vi "Fluence in multiple areas.vi"(0 "Analyze Fluence in":refnum<class "Analyze Fluence.lvclass">, 5 "Image in":T2, 7 "Energy":dbl[unit], 11 "error in (no error)":errorcluster) -> (4 "Analyze Fluence out":refnum<class "Analyze Fluence.lvclass">, 6 "Image Dst Out":T2, 8 "Max Fluence J/cm^2":dbl[unit], 10 "fluence infos":T3[](array[typedef]), 15 "error out":errorcluster)   [LabVIEW 2014, in "Analyze.lvlib" / "Analyze Fluence.lvclass"]
uses:
  Analyze Fluence.lvclass
  Fluence Info.ctl
  <vilib>/vision/Image Controls.llb/IMAQ Image.ctl
  Analyze Parameter/Analyze Parameter Fluence/Analyze Parameter Fluence.lvclass
  Analyze Fluence.lvclass/Analyze Fluence.ctl
  <vilib>/vision/NI_Vision_Development_Module.lvlib
  Analyze BaseClass/Analyze BaseClass/Analyze BaseClass.lvclass
panel:
  in  "ROI Descriptor out":T1 {"Contours"."Type" items=["No Selection", "Point", "Line", "Rectangle", "Oval", "Polygon", "Freehand Region", "Annulus", "Unused2", "Unused3", "Broken Line", "Freehand Line", "Rotated Rectangle"]}
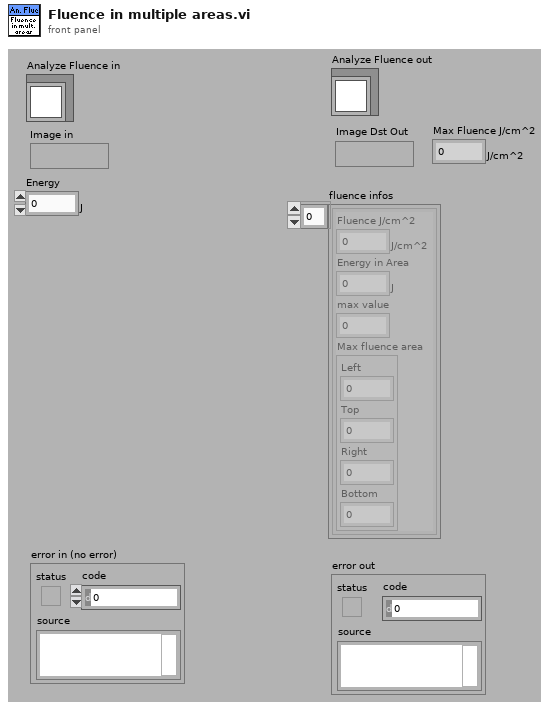
[diagram p1: front panel]
types:
  T1 = typedef "ROI Descriptor" = cluster{"Global Rectangle":i32[], "Contours":cluster{"ID":enum32{"External", "Internal"}, "Type":u32, "Coordinates":i32[]}[]}
  T2 = typedef "IMAQ Image.ctl" = refnum<image>
  T3 = typedef "Analyze.lvlib/Analyze Fluence.lvclass/Fluence Info.ctl" = cluster{"Fluence J/cm^2":dbl[unit], "Energy in Area":dbl[unit], "max value":i64, "Max fluence area":cluster{"Left":i32, "Top":i32, "Right":i32, "Bottom":i32}}
  T4 = typedef "IMAQ Rectangle" = cluster{"Left":i32, "Top":i32, "Right":i32, "Bottom":i32, "Rotation":dbl}
  T5 = typedef "Image Type" = u32
  T6 = cluster{"Left":i32, "Top":i32, "Right":i32, "Bottom":i32}
  T7 = cluster{"Fluence J/cm^2":dbl[unit], "Energy in Area":dbl[unit], "max value":i64, "Max fluence area":cluster{"Left":i32, "Top":i32, "Right":i32, "Bottom":i32}}
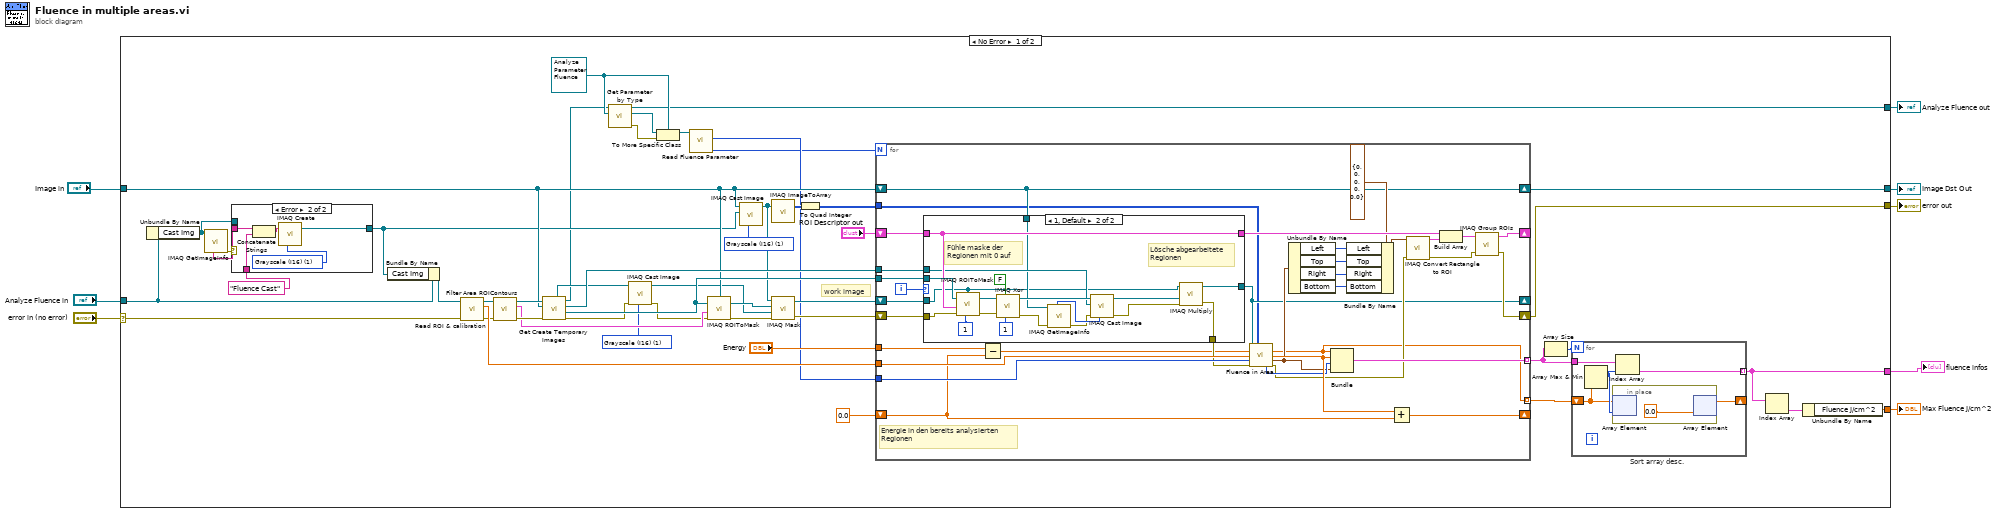
[diagram p0: block diagram]
diagram:
  n1 = case shown="No Error" "error in (no error)" {
    selector: "error in (no error)" -> [w9 w128]
    tunnel: [w54 _] -> w8
    tunnel: [w53 w126] -> w7
    tunnel: [w52 w128] -> w6
    tunnel: "Image in" -> [w38 w126]
    tunnel: "Analyze Fluence in" -> [w35 w127]
    tunnel: [w12 w127] -> w3
    tunnel: [w10 _] -> w2
    frame No Error {
      w15 = refnum<class "Analyze Parameter Fluence.lvclass"> refnum ("Parameter")
      w26 = T5 1 items=["Grayscale (U8)", "Grayscale (I16)", "Grayscale (SGL)", "Complex (CSG)", "RGB (U32)", "HSL (U32)", "RGB (U64)", "Grayscale (U16)"] ("Image Type")
      w36 = T5 1 items=["Grayscale (U8)", "Grayscale (I16)", "Grayscale (SGL)", "Complex (CSG)", "RGB (U32)", "HSL (U32)", "RGB (U64)", "Grayscale (U16)"] ("Image Type")
      # "work image"
      n2 = Unbundle By Name(w35) -> ("Cast Img"=w31:T2)
      n3 = call "IMAQ GetImageInfo"("Image"=w31) -> ("error out"=w34:errorcluster, "Image Name"=w33:string)  [unwired: 3 in, 6 out]
      n4 = case shown="Error" w34 {
        tunnel: w33 -> [_ w124]
        tunnel: "Fluence Cast" -> [_ w122]
        tunnel: [w120 w121] -> w29
        tunnel: w31 -> [w120 _]
        frame No Error {
        }
        frame Error {
          w125 = T5 1 items=["Grayscale (U8)", "Grayscale (I16)", "Grayscale (SGL)", "Complex (CSG)", "RGB (U32)", "HSL (U32)", "RGB (U64)", "Grayscale (U16)"] ("Image Type")
          n5 = Concatenate Strings(w124, w122) -> (w123:string)
          n6 = call "IMAQ Create"("Image Name"=w123, "Image Type"=w125) -> ("New Image"=w121:T2)  [unwired: 3 in, 1 out]
        }
      }
      n7 = Bundle By Name(cluster=w35, "Cast Img"=w29) -> (w30:refnum<class "Analyze Fluence.lvclass">)
      n8 = call-dynamic "Read ROI & calibration.vi"("error in (no error)"=w9, "Analyze BaseClass in"=w30) -> ("error out"=w46:errorcluster, "calibration mm/px"=w49:dbl[unit], "Analyze BaseClass out"=w48:refnum<class "Analyze Fluence.lvclass">)  [unwired: 6 in, 1 out]
      n9 = call-dynamic "Filter Area ROIContours.vi"("error in (no error)"=w46, "Analyze BaseClass in"=w48) -> ("error out"=w45:errorcluster, "ROI of Area type"=w39:T1, "Analyze BaseClass out"=w47:refnum<class "Analyze Fluence.lvclass">)  [unwired: 7 in]
      n10 = call-dynamic "Get Create Temporary Images.vi"("error in (no error)"=w45, "Image in"=w38, "Analyze BaseClass in"=w47) -> ("error out"=w25:errorcluster, "image mask"=w50:T2, "work image"=w42:T2, "Analyze BaseClass out"=w13:refnum<class "Analyze Fluence.lvclass">, "masked image"=w28:T2)  [unwired: 4 in]
      n11 = call "Get Parameter by Type.vi"("Parameter Type"=w15, "Analyze BaseClass in"=w13) -> ("error out"=w16:errorcluster, "Parameter"=w14:refnum<class "Analyze Parameter Base.lvclass">, "Analyze BaseClass out"=w12:refnum<class "Analyze Fluence.lvclass">)  [unwired: 6 in, 1 out]
      n12 = call "IMAQ Cast Image"("Image Type"=w26, "error in (no error)"=w25, "Image Src"=w28) -> ("error out"=w24:errorcluster, "Image Dst Out"=w27:T2)  [unwired: 7 in]
      n13 = To More Specific Class(target class=w15, reference=w14, error in=w16) -> (specific class reference=w11:refnum<class "Analyze Parameter Fluence.lvclass">)  [unwired: 1 out]
      n14 = call "Read Fluence Parameter.vi"("Analyze Parameter Fluence in"=w11) -> ("#of Areas"=w17:i32, "Size of region (px)"=w18:i32)  [unwired: 7 in, 2 out]
      n15 = call "IMAQ ROIToMask"("error in (no error)"=w24, "ROI Descriptor"=w39, "Image"=w50, "Image Model"=w38) -> ("error out"=w51:errorcluster, "Image Out"=w56:T2)  [unwired: 2 in, 1 out]
      n16 = call "IMAQ Cast Image"("Image Type"=w36, "Image Dst"=w29, "Image Src"=w38) -> ("Image Dst Out"=w37:T2)  [unwired: 7 in, 1 out]
      n17 = call "IMAQ ImageToArray"("Image"=w37) -> ("Image Pixels (I16)"=w41:i16[][])  [unwired: 3 in, 4 out]
      n18 = call "IMAQ Mask"("error in (no error)"=w51, "Image Dst"=w27, "Image Mask"=w56, "Image Src"=w37) -> ("error out"=w43:errorcluster, "Image Dst Out"=w44:T2)  [unwired: 1 in]
      n19 = To Quad Integer(1:w41) -> (0:w40:i64[][])
      n20 = for {
        N: w17 -> [_]
        tunnel: "Energy" -> [w91]
        tunnel: w49 -> [w90]
        tunnel: w18 -> [w89]
        shift-right: [w88] -> _
        shift-left: "ROI Descriptor out" -> [w82]
        tunnel: w50 -> [w87]
        tunnel: w42 -> [w85]
        shift-right: [w61] -> _
        shift-left: w44 -> [w62]
        shift-right: [w65] -> w52
        shift-left: w43 -> [w86]
        shift-right: [w84] -> _
        shift-left: dbl[unit] 0.0 ("Energy in Area") -> [w83]
        tunnel: [w63] -> w20 mode=indexing
        shift-right: [w59] -> w53
        shift-left: w38 -> [w59]
        tunnel: [w66] -> w21 mode=indexing
        tunnel: w40 -> [w58]
        i -> [w69]
        # "Energie in den bereits analysierten \nRegionen"
        n21 = case shown="1, Default" w69 {
          tunnel: w87 -> [_ w109]
          tunnel: w86 -> [w94 w108]
          tunnel: w85 -> [_ w97]
          tunnel: w62 -> [w93 w95]
          tunnel: w82 -> [w92 w101]
          tunnel: [w94 w111] -> w74
          tunnel: [w93 w110] -> w61
          tunnel: [w92 w101] -> w67
          tunnel: w59 -> [_ w96]
          frame 0 {
          }
          frame 1, Default {
            # "Lösche abgearbeitete\nRegionen"
            # "Fühle maske der\nRegionen mit 0 auf"
            n22 = call "IMAQ ROIToMask"("error in (no error)"=w108, "ROI Descriptor"=w101, "Filling Value (255)"=1 ("Background Value (0)"), "Image"=w109, "Image Model"=w95) -> ("error out"=w104:errorcluster, "Image Out"=w103:T2)  [unwired: 1 in, 1 out]
            n23 = call "IMAQ Xor"("Constant"=1, "Xor/Xnor (Xor)"=FALSE ("And/Nand (And)"), "error in (no error)"=w104, "Image Src A"=w103) -> ("error out"=w99:errorcluster, "Image Dst Out"=w102:T2)  [unwired: 6 in]
            n24 = call "IMAQ GetImageInfo"("error in (no error)"=w99, "Image"=w96) -> ("error out"=w98:errorcluster, "Image Type"=w100:T5)  [unwired: 2 in, 6 out]
            n25 = call "IMAQ Cast Image"("Image Type"=w100, "error in (no error)"=w98, "Image Dst"=w97, "Image Src"=w102) -> ("error out"=w112:errorcluster, "Image Dst Out"=w113:T2)  [unwired: 6 in]
            n26 = call "IMAQ Multiply"("Image Src A"=w95, "Image Src B"=w113, "error in (no error)"=w112) -> ("Image Dst Out"=w110:T2, "error out"=w111:errorcluster)  [unwired: 4 in]
          }
        }
        n27 = Subtract(x=w91, y=w83) -> (x-y=w73:dbl[unit])
        n28 = call "Fluence in Area.vi"("Masked Image (I16only)"=w61, "Origin Image"=w58, "Energie"=w73, "calibration mm/px"=w90, "Size of region"=w89, "error in (no error)"=w74) -> ("Fluence J/cm^2"=w63:dbl[unit], "Energy in Area"=w72:dbl[unit], "Max fluence area"=w70:T6, "max value"=w71:i64, "error out"=w64:errorcluster)  [unwired: 5 in]
        n29 = Unbundle By Name(w70) -> ("Left"=w78:i32, "Top"=w79:i32, "Right"=w80:i32, "Bottom"=w81:i32)
        n30 = Bundle("Fluence J/cm^2"=w63, "Energy in Area"=w72, "max value"=w71, "Max fluence area"=w70) -> (w66:T7)  [unwired: 1 in]
        n31 = Bundle By Name(cluster=T4 {"Left"=0, "Top"=0, "Right"=0, "Bottom"=0, "Rotation"=0.0} ("Rectangle"), "Left"=w78, "Top"=w79, "Right"=w80, "Bottom"=w81) -> (w77:T4)
        n32 = Add(x=w72, y=w83) -> (x+y=w84:dbl[unit])
        n33 = call "IMAQ Convert Rectangle to ROI"("error in (no error)"=w64, "Rectangle"=w77) -> ("error out"=w68:errorcluster, "ROI Descriptor"=w76:T1)  [unwired: 7 in]
        n34 = Build Array(w67, w76) -> (w75:T1[])
        n35 = call "IMAQ Group ROIs"("error in (no error)"=w68, "ROI Descriptors"=w75) -> ("error out"=w65:errorcluster, "ROI Descriptor out"=w88:T1)  [unwired: 2 in]
      }
      n36 = Array Size(array=w21) -> (size(s)=w22:i32)
      n37 = for "Sort array desc." {
        N: w22 -> [_]
        shift-right: [w114] -> _
        shift-left: w20 -> [w115]
        tunnel: w21 -> [w118]
        tunnel: [w117] -> w10 mode=indexing
        n38 = Array Max & Min(array=w115) -> (max index (indices)=w116:i32)  [unwired: 3 out]
        n39 = in-place {
          n40 = in-place-array #1(w115, w116) -> ()  [unwired: 1 out]
          n41 = in-place-array #1(dbl[unit] 0.0 ("element")) -> (w114:dbl[unit][])  [unwired: 1 out]
        }
        n42 = Index Array(array=w118, index=w116) -> (element=w117:T7)
      }
      n43 = Index Array(array=w10) -> (element=w55:T7)  [unwired: 1 in]
      n44 = Unbundle By Name(w55) -> ("Fluence J/cm^2"=w54:dbl[unit])
    }
    frame Error {
    }
  }
  "error out" <- w6
  "Image Dst Out" <- w7
  "Max Fluence J/cm^2" <- w8
  "Analyze Fluence out" <- w3
  "fluence infos" <- w2
